vi "ReCalc - Enable_AFR_EGT_Graph (SubVI).vi"(0 "Leistungsgraph":refnum<vi>, 1 "AFR EGT":bool, 7 "Höhe Leistungs-Graph":u32, 9 "AFR EGT Gaph":refnum<vi>, 14 "Skalierungsfaktor Leistungsgraph":dbl) -> ()   [LabVIEW 2014]
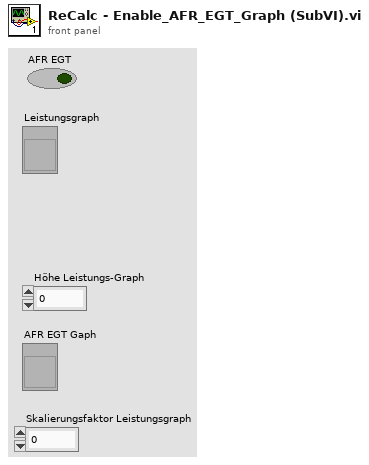
[diagram p1: front panel]
types:
  T1 = typedef "LVRangeTypeDef.ctl" = cluster{"Minimum":dbl, "Maximum":dbl, "Increment":dbl, "Minor Increment":dbl, "Start":dbl}
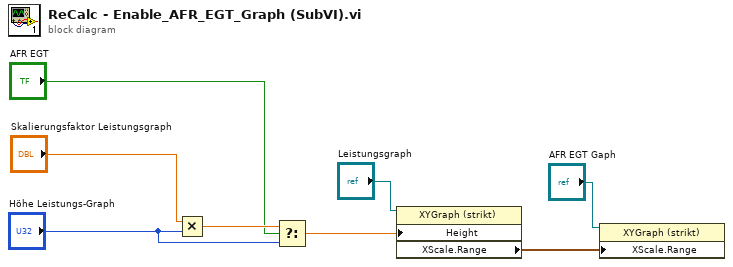
[diagram p0: block diagram]
diagram:
  n1 = Multiply(x="Skalierungsfaktor Leistungsgraph", y="Höhe Leistungs-Graph") -> (x*y=w8:dbl)
  n2 = Select(t=w8, s="AFR EGT", f="Höhe Leistungs-Graph") -> (s? t:f=w5:dbl)
  n3 = property on="Eigenschaftsknoten" class="XYGraph (strikt)"(reference="Leistungsgraph", "Height"=w5) -> ("XScale.Range"=w3:T1)  [unwired: 1 in, 2 out]
  n4 = property on="Eigenschaftsknoten" class="XYGraph (strikt)"(reference="AFR EGT Gaph", "XScale.Range"=w3) -> ()  [unwired: 1 in, 2 out]
